vi "Get Top Elements By Type.vi"(7 "Other Refnum":refnum<vi>, 8 "error in (no error)":errorcluster, 10 "type":T1="ForLoop", 11 "VI in":refnum<vi>) -> (0 "error out":errorcluster, 2 "# of Refs":i32, 3 "References":refnum<vi>[](array[refnum]))   [LabVIEW 2014]
uses:
  types/Entities.ctl
  <vilib>/Utility/traverseref.llb/TRef TravTarget.ctl
  <vilib>/Utility/traverseref.llb/VI Scripting - Traverse.lvlib
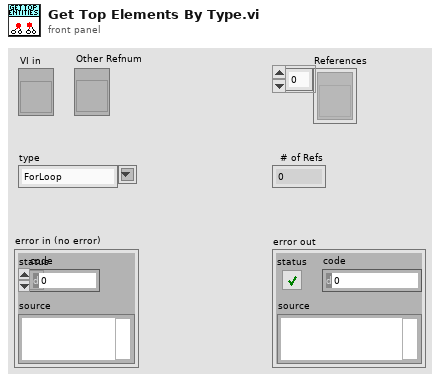
[diagram p1: front panel]
types:
  T1 = typedef "Entities.ctl" = string
  T2 = typedef "TRef TravTarget.ctl" = enum16{"FP", "BD", "Other"}
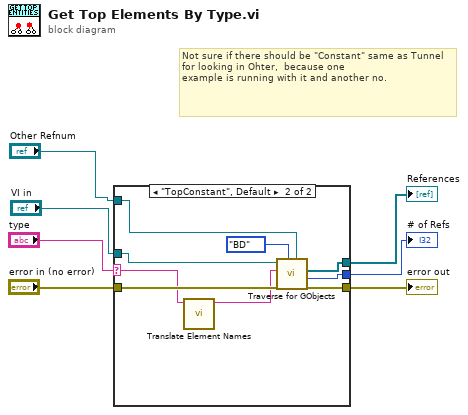
[diagram p0: block diagram]
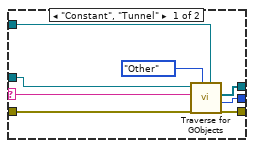
[diagram p2: hidden frame]
diagram:
  # "Not sure if there should be \"Constant\" same as Tunnel for looking in Ohter,  because one\nexample is running with it and another no."
  n1 = case shown="\"TopConstant\", Default" "type" {
    selector: "type" -> [w12 w17]
    tunnel: "VI in" -> [w11 w24]
    tunnel: [w13 w23] -> w6
    tunnel: [w10 w22] -> w5
    tunnel: "error in (no error)" -> [w14 w20]
    tunnel: [w9 w19] -> w2
    tunnel: "Other Refnum" -> [w8 w18]
    frame "Constant", "Tunnel" {
      n2 = call <vilib>:"Traverse for GObjects.vi"("Other Refnum"=w8, "Traverse Target"=TRef_TravTarget."Other", "error in (no error)"=w14, "Class Name"=w12, "VI Refnum"=w11) -> ("error out"=w13:errorcluster, "# of Refs"=w9:i32, "References"=w10:refnum<vi>[])  [unwired: 3 in, 1 out]
    }
    frame "TopConstant", Default {
      n3 = call "Translate Element Names.vi"("Element Name"=w17) -> ("Translated Element Name to Basic Name"=w16:string)  [unwired: 10 in]
      n4 = call <vilib>:"Traverse for GObjects.vi"("Other Refnum"=w18, "Traverse Target"=TRef_TravTarget."BD", "error in (no error)"=w20, "Class Name"=w16, "VI Refnum"=w24) -> ("error out"=w23:errorcluster, "# of Refs"=w19:i32, "References"=w22:refnum<vi>[])  [unwired: 3 in, 1 out]
    }
  }
  "error out" <- w6
  "References" <- w5
  "# of Refs" <- w2
